vi "Notify State.vi"(8 "error in (no error)":errorcluster, 11 "_State Machine Actor in":refnum<class "_State Machine Actor.lvclass">) -> (0 "error out":errorcluster, 3 "_State Machine Actor out":refnum<class "_State Machine Actor.lvclass">)   [LabVIEW 2024]
uses:
  _State Machine Actor.lvclass
  _State Machine Actor.lvclass/_State Machine Actor.ctl
  Context/Context/Context.lvclass
  C:/Program Files (x86)/National Instruments/LabVIEW 2024/vi.lib/ActorFramework/Actor/Actor.lvclass
  C:/Users/uspoaotto/OneDrive - Oregon Tool/Desktop/working copies/stateMachineActor/src/_State Machine Actor/_State Machine Actor/_State Machine Actor.lvclass
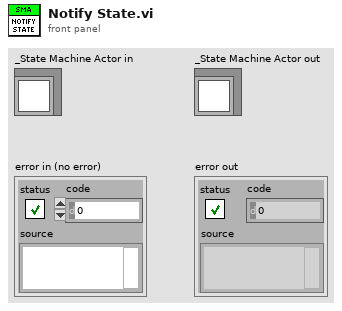
[diagram p1: front panel]
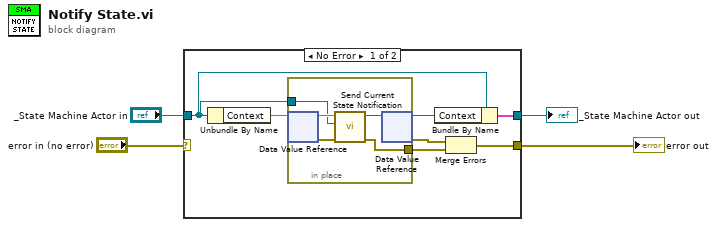
[diagram p0: block diagram]
diagram:
  n1 = case shown="No Error" "error in (no error)" {
    selector: "error in (no error)" -> [_ w18]
    tunnel: [w5 w18] -> w3
    tunnel: [w9 w17] -> w1
    tunnel: "_State Machine Actor in" -> [w10 w17]
    frame No Error {
      n2 = Unbundle By Name(w10) -> ("Context"=w11)
      n3 = in-place {
        in-place-border: w10 -> [w15]
        in-place-border: [w12] -> w6
        n4 = in-place-dvr #1(w11) -> (w16:dbl, w13:errorcluster)
        n5 = call "Send Current State Notification.vi"("error in (no error)"=w13, "State"=w15, "Context in"=w16) -> ("error out"=w12:errorcluster, "Context out"=w14:refnum<class "Context.lvclass">)  [unwired: 7 in]
        n6 = in-place-dvr #1(w14) -> (w8:refnum<data-value>, w7:errorcluster)
      }
      n7 = Bundle By Name(cluster=w10, "Context"=w8) -> (w9:cluster{})
      n8 = Merge Errors(w7, w6) -> (w5:errorcluster)
    }
    frame Error {
    }
  }
  "error out" <- w3
  "_State Machine Actor out" <- w1
